vi "SR830 single initalize.vi"(0 "VISA引用句柄输入":refnum<visa-resource-name>, 1 "输入信号":T3, 2 "滤波设置":T1, 5 "open":bool, 7 "参考信号":T2, 9 "量程":enum16{"量程每次测量会判定", "量程不变为设定值"}(ring), 11 "error in (no error)":errorcluster, 12 "ID Query (True)":bool, 13 "Reset (True)":bool, 14 "Sensitivity (-1: Auto gain)":i16) -> (15 "错误输出":cluster{"status":bool, "code":i32, string})   [LabVIEW 2019, in "SubVI.lvlib"]
uses:
  SubVI.lvlib
  lib/Stanford Research 830/Public/Data/Read (All Parameters).vi
  lib/Stanford Research 830/Stanford Research 830.lvlib
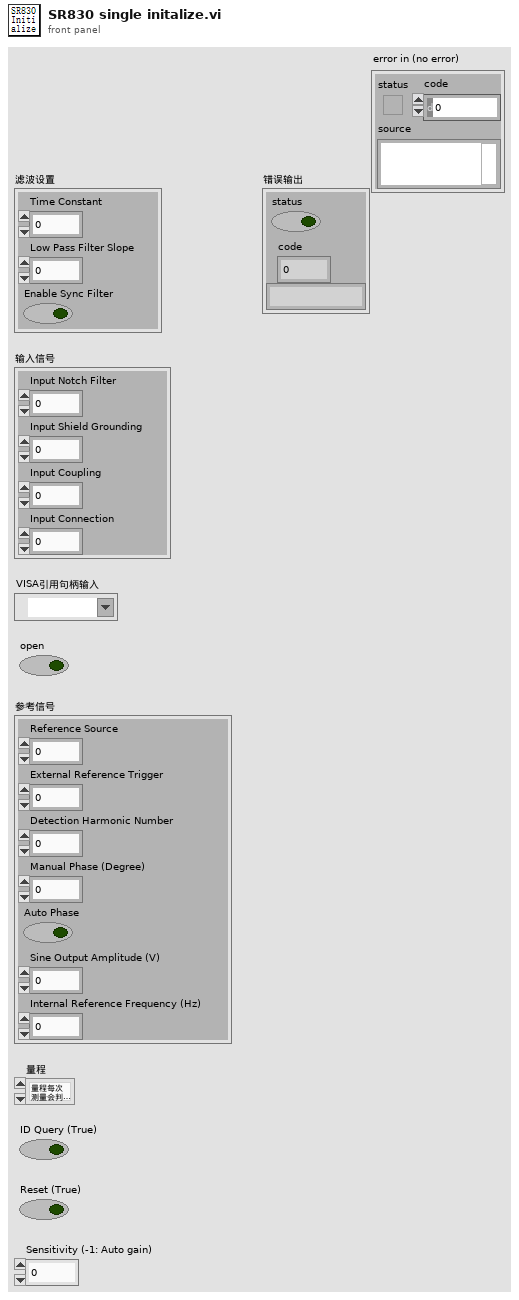
[diagram p1: front panel]
types:
  T1 = cluster{"Time Constant ":u16, "Low Pass Filter Slope ":u16, "Enable Sync Filter ":bool}
  T2 = cluster{"Reference Source":u16, "External Reference Trigger  ":u16, "Detection Harmonic Number ":dbl, "Manual Phase (Degree)":dbl, "Auto Phase ":bool, "Sine Output Amplitude (V)":dbl, "Internal Reference Frequency (Hz)":dbl}
  T3 = cluster{"Input Notch Filter ":u16, "Input Shield Grounding":u16, "Input Coupling ":u16, "Input Connection  ":u16}
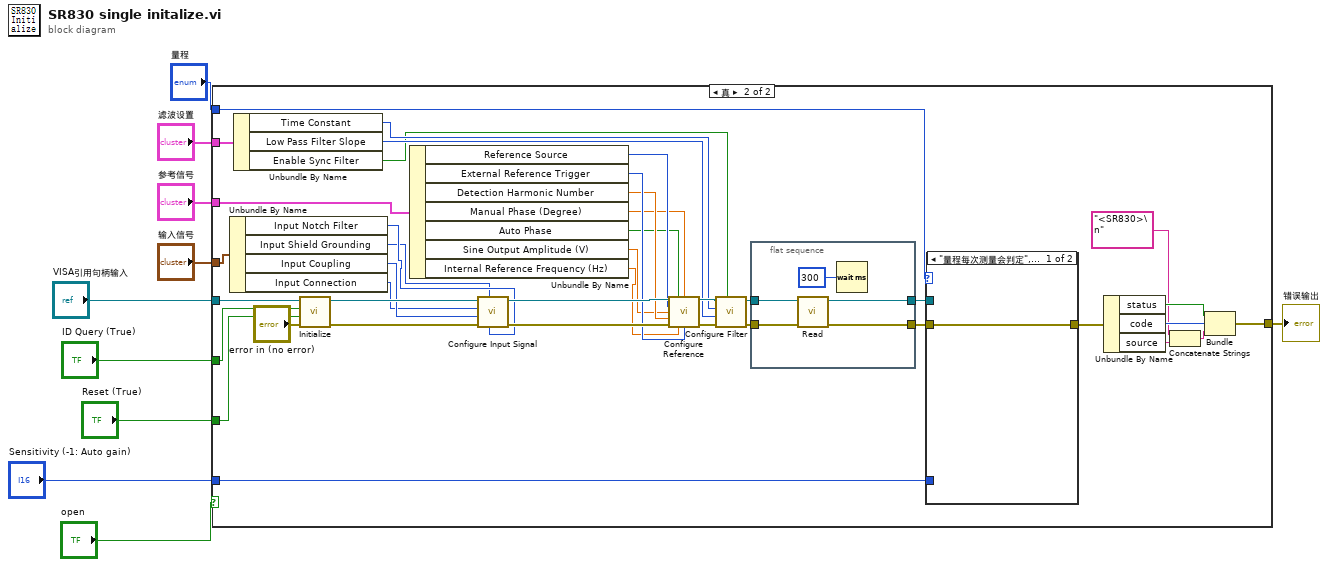
[diagram p0: block diagram]
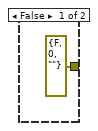
[diagram p2: hidden frame]
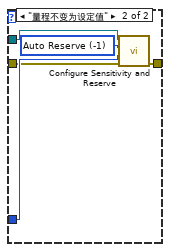
[diagram p3: hidden frame]
diagram:
  n1 = case shown="真" "open" {
    tunnel: "VISA引用句柄输入" -> [_ w51]
    tunnel: "ID Query (True)" -> [_ w42]
    tunnel: "Reset (True)" -> [_ w41]
    tunnel: [cluster{"status":bool, "code":i32, string} {"status"=FALSE, "code"=0, ""} w28] -> w5
    tunnel: "滤波设置" -> [_ w24]
    tunnel: "参考信号" -> [_ w23]
    tunnel: "输入信号" -> [_ w22]
    tunnel: "量程" -> [_ w17]
    tunnel: "Sensitivity (-1: Auto gain)" -> [_ w16]
    frame False {
    }
    frame True {
      n2 = Unbundle By Name(w22) -> ("Input Notch Filter"=w21:u16, "Input Shield Grounding"=w20:u16, "Input Coupling"=w19:u16, "Input Connection"=w18:u16)
      n3 = Unbundle By Name(w24) -> ("Time Constant"=w27:u16, "Low Pass Filter Slope"=w26:u16, "Enable Sync Filter"=w25:bool)
      n4 = call "Initialize.vi"("error in (no error)"="error in (no error)", "Reset (True)"=w41, "ID Query (True)"=w42, "VISA resource name"=w51) -> ("error out"=w49:errorcluster, "VISA resource name out"=w50:refnum<visa-resource-name>)  [unwired: 6 in]
      n5 = Unbundle By Name(w23) -> ("Reference Source"=w40:u16, "External Reference Trigger"=w39:u16, "Detection Harmonic Number"=w38:dbl, "Manual Phase (Degree)"=w37:dbl, "Auto Phase"=w36:bool, "Sine Output Amplitude (V)"=w35:dbl, "Internal Reference Frequency (Hz)"=w34:dbl)
      n6 = call "Configure Input Signal.vi"("Input Notch Filter (0: None)"=w21, "Input Shield Grounding (0: Float)"=w20, "error in (no error)"=w49, "Input Coupling (0: AC)"=w19, "Input Connection (0: Single-Ended Voltage)"=w18, "VISA resource name"=w50) -> ("error out"=w47:errorcluster, "VISA resource name out"=w48:refnum<visa-resource-name>)  [unwired: 4 in]
      n7 = call "Configure Reference.vi"("VISA resource name"=w48, "Auto Phase (T: Enabled)"=w36, "Manual Phase (0 Degree)"=w37, "Reference Source (1: Internal)"=w40, "Sine Output Amplitude (1 V)"=w35, "Detection Harmonic Number (1)"=w38, "error in (no error)"=w47, "Internal Reference Frequency (1000 Hz)"=w34, "External Reference Trigger (0: Sine Zero Crossing)"=w39) -> ("VISA resource name out"=w46:refnum<visa-resource-name>, "error out"=w45:errorcluster)  [unwired: 5 in]
      n8 = call "Configure Filter.vi"("Enable Sync Filter (F: Disable)"=w25, "error in (no error)"=w45, "Low Pass Filter Slope (1: 12dB/oct)"=w26, "Time Constant (8: 100ms)"=w27, "VISA resource name"=w46) -> ("error out"=w43:errorcluster, "VISA resource name out"=w44:refnum<visa-resource-name>)  [unwired: 5 in]
      n9 = flat-sequence {
        tunnel: [w62] -> w15
        tunnel: w44 -> [w61]
        tunnel: w43 -> [w60]
        tunnel: [w58] -> w14
        frame #0 {
          n10 = call-poly "Read.vi"("error in (no error)"=w60, "VISA resource name"=w61) -> ("error out"=w58:errorcluster, "VISA resource name out"=w62:refnum<visa-resource-name>)  [unwired: 7 in, 1 out]
          n11 = Wait (ms)(milliseconds to wait=u32 300 ("等待时间（毫秒）")) -> ()  [unwired: 1 out]
        }
      }
      n12 = case shown="\"量程每次测量会判定\", 默认" w17 {
        tunnel: w16 -> [_ w56]
        tunnel: w15 -> [_ w55]
        tunnel: w14 -> [w52 w54]
        tunnel: [w52 w53] -> w13
        frame "量程每次测量会判定", Default {
        }
        frame "量程不变为设定值" {
          w57 = i16 -1 items=["Auto Reserve"=-1, "High Reserve"=0, "Normal"=1, "Low Noise"=2] ("Dynamic Reserve (-1: Auto Reserve)")
          n13 = call "Configure Sensitivity and Reserve.vi"("error in (no error)"=w54, "Sensitivity (-1: Auto gain)"=w56, "Dynamic Reserve (-1: Auto Reserve)"=w57, "VISA resource name"=w55) -> ("error out"=w53:errorcluster)  [unwired: 6 in, 1 out]
        }
      }
      n14 = Unbundle By Name(w13) -> ("status"=w31:bool, "code"=w32:i32, "source"=w30:string)
      n15 = Concatenate Strings("<SR830>\n", w30) -> (w33:string)
      n16 = Bundle("status"=w31, "code"=w32, w33) -> (w28:cluster{"status":bool, "code":i32, string})  [unwired: 1 in]
    }
  }
  "错误输出" <- w5
